vi "Build Scalar Group Channels.vi"(6 "error in (no error)":errorcluster, 7 "scalar channel in":T2 {"Data Type" format="%.0x"}, 9 "item ref in":T1 format="%.0x") -> (0 "error out":errorcluster, 3 "built channels out":T4[](array[typedef]) {"Item Ref" format="%.0x"})   [LabVIEW 2018, in "FPGA Addon System Explorer.lvlib"]
uses:
  FPGA Addon System Explorer.lvlib
  Types/Output Scalar.ctl
  Addon Shared/Types/Data Type.ctl
  <vilib>/NI Veristand/Custom Device API/Custom Device Item Ref.ctl
  Addon Shared/Types/Register Information.ctl
  Addon Shared/FPGA Addon Shared.lvlib
  <vilib>/NI Veristand/Custom Device Tools/Custom Device Utility Library/Custom Device Utility Library.lvlib
  <vilib>/NI Veristand/Custom Device API/Custom Device API.lvlib
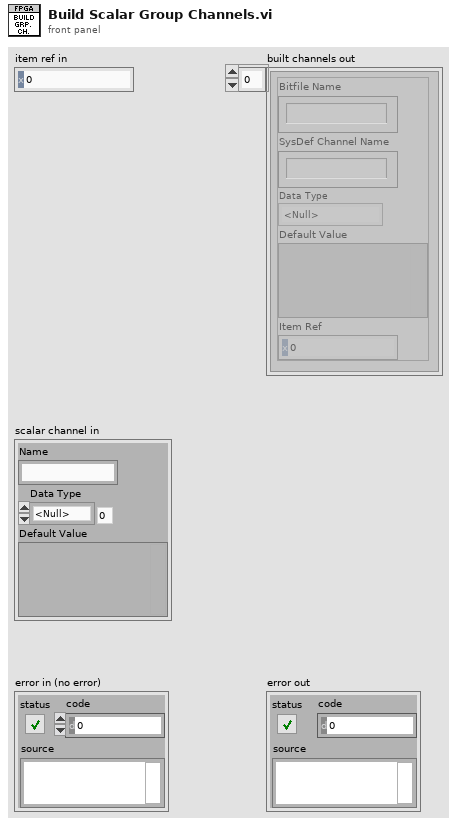
[diagram p1: front panel]
types:
  T1 = typedef "Custom Device API.lvlib/Custom Device Item Ref.ctl" = u64
  T2 = typedef "FPGA Addon Shared.lvlib/Register Information.ctl" = cluster{"Name":string, "Data Type":T3, "Default Value":variant}
  T3 = typedef "FPGA Addon Shared.lvlib/Data Type.ctl" = enum8{"<Null>", "I8", "I16", "I32", "I64", "U8", "U16", "U32", "U64", "SGL", "Boolean", "Analog PWM In Settings", "Analog PWM In", "Digital PWM In Settings", "Digital PWM In", "Digital PWM Out", "Sine Out", "FXP+/-24.5", "FXP+/-16.5", "FXP+/-32.8", "FXP+/-64.32", "FXP+/-16.7", "FXP+/-20.5", "FXP+/-27.5", "FXP+/-32.16", "FXP+16.3", "FXP+18.3", "Digital Static In", "Digital Static Out", "Digital Static In Settings", "Digital WSS Out", "Quad Encoder Settings", "Quad Encoder In", "Group"}
  T4 = typedef "FPGA Addon System Explorer.lvlib/Output Scalar.ctl" = cluster{"Bitfile Name":string, "SysDef Channel Name":string, "Data Type":T3, "Default Value":variant, "Item Ref":T1}
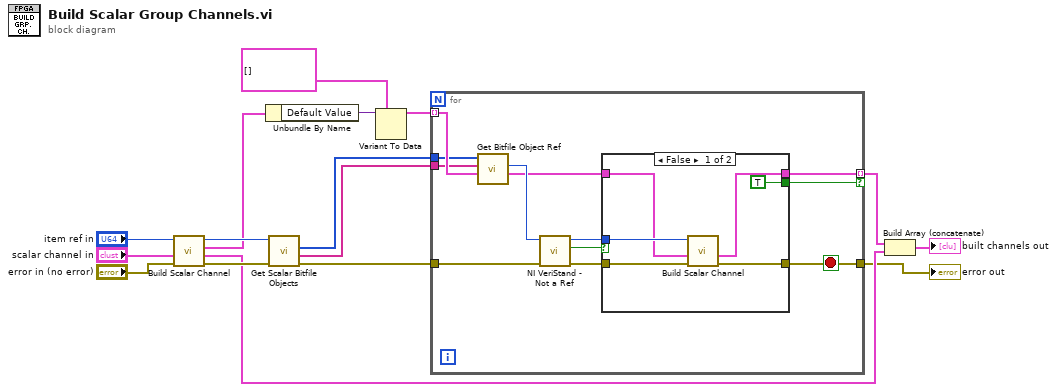
[diagram p0: block diagram]
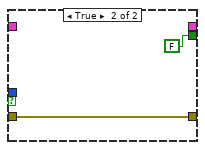
[diagram p2: hidden frame]
diagram:
  n1 = call "Build Scalar Channel.vi"("error in (no error)"="error in (no error)", "scalar channel in"="scalar channel in", "item ref in"="item ref in") -> ("error out"=w14:errorcluster, "built scalar channel out"=w13:T4, "scalar channel out"=w5:T2, "item ref out"=w7:T1)  [unwired: 5 in]
  n2 = Unbundle By Name(w5) -> ("Default Value"=w6:variant)
  n3 = call "Get Scalar Bitfile Objects.vi"("error in"=w14, "item ref in"=w7) -> ("error out"=w15:errorcluster, "bitfile object names"=w10:string[], "section children refs"=w8:T1[])  [unwired: 6 in, 1 out]
  n4 = Variant To Data(type=T2[] [], Variant=w6) -> (data=w9:T2[])  [unwired: 1 in, 1 out]
  n5 = for {
    tunnel: w8 -> [w26]
    tunnel: w9 -> [w28] mode=indexing
    tunnel: w10 -> [w27]
    tunnel: w15 -> [w24]
    tunnel: [w17] -> w11
    tunnel: [w19] -> w12 mode=indexing if=w18
    stop <- w17 stop-if-true
    n6 = call "Get Bitfile Object Ref.vi"("scalar channel in"=w28, "bitfile object names"=w27, "section children refs in"=w26) -> ("scalar channel out"=w20:T2, "item ref out"=w25:T1)  [unwired: 6 in, 1 out]
    n7 = call <vilib>:"NI VeriStand - Not a Ref.vi"("error in (no error)"=w24, "Item Ref"=w25) -> ("error out"=w22:errorcluster, "Not a Ref"=w23:bool, "Item Ref out"=w21:T1)  [unwired: 7 in]
    n8 = case shown="False" w23 {
      tunnel: w22 -> [w34 w35]
      tunnel: [w33 w35] -> w17
      tunnel: w21 -> [w32 _]
      tunnel: w20 -> [w29 _]
      tunnel: [w31 _] -> w19
      tunnel: [TRUE FALSE] -> w18
      frame False {
        n9 = call "Build Scalar Channel.vi"("error in (no error)"=w34, "scalar channel in"=w29, "item ref in"=w32) -> ("error out"=w33:errorcluster, "built scalar channel out"=w31:T4)  [unwired: 5 in, 2 out]
      }
      frame True {
      }
    }
  }
  "error out" <- w11
  n10 = Build Array (concatenate)(w12, w13) -> (→"built channels out":T4[])
